vi "Launcher.vi"() -> ()   [LabVIEW 2019, in "Aplicacion.lvclass"]
uses:
  Aplicacion.lvclass
  Pruebas/AjustesPrevios/AjustesPrevios.lvclass
  Equipo/Equipo/Equipo.lvclass
  Equipo/Fabrica de Equipos/Fabrica de Equipos.lvclass
panel:
  in  "Certificado":bool
  in  "Salir":bool
  in  "Ensayos":bool
  in  "Configuraciones":bool
  in  "Usuarios":bool
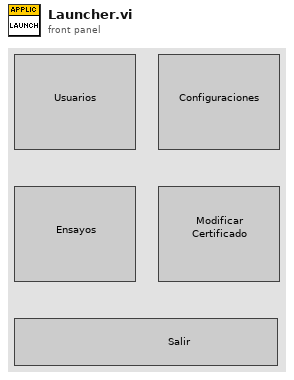
[diagram p1: front panel]
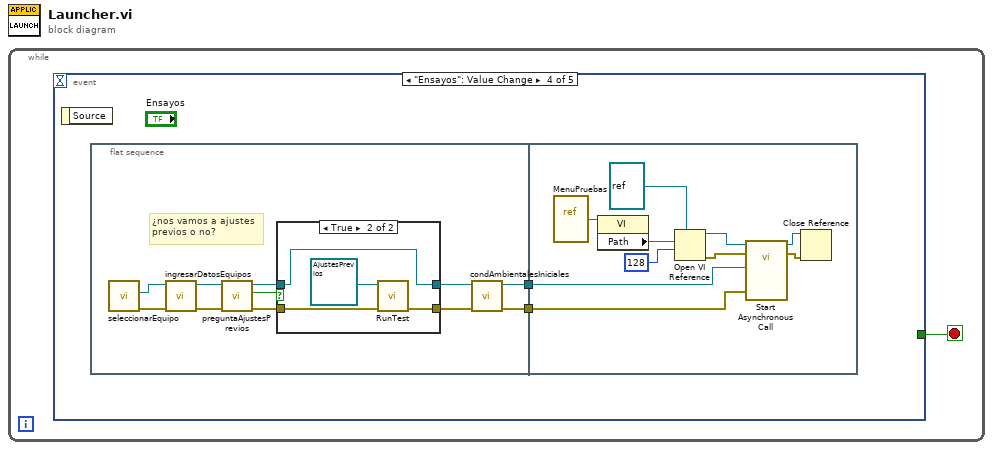
[diagram p0: block diagram]
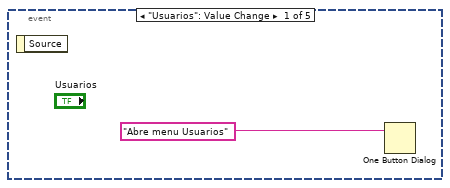
[diagram p2: hidden frame]
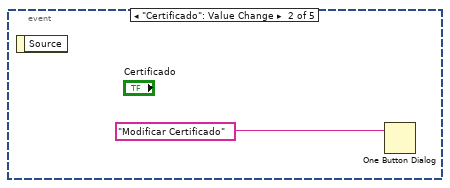
[diagram p3: hidden frame]
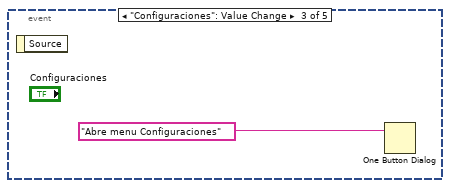
[diagram p4: hidden frame]
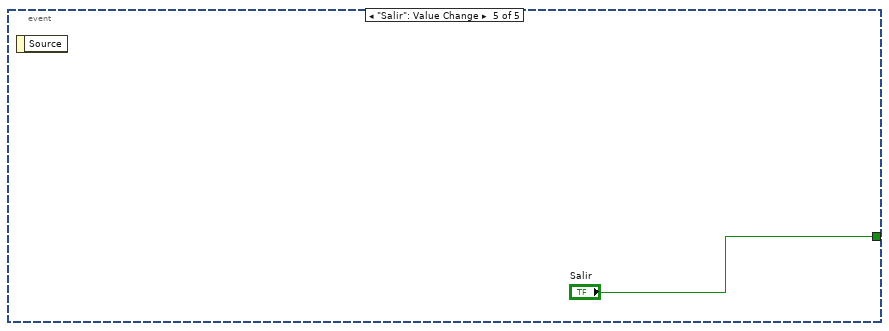
[diagram p6: hidden frame]
diagram:
  n1 = while {
    stop <- w1 stop-if-true
    n2 = event shown="[3] \"Ensayos\": Value Change" {
      selector: _ -> [_ _ _ _ _]
      dyn-events: _ -> [_ _ _ _ _]
      timeout: _ -> [_ _ _ _ _]
      tunnel: [_ _ _ _ "Salir"] -> w1
      event "Usuarios": Value Change {
        n3 = event-data() -> ()  [unwired: 1 in, 1 out]
        n4 = One Button Dialog(message="Abre menu Usuarios") -> ()  [unwired: 1 in, 1 out]
      }
      event "Certificado": Value Change {
        n5 = event-data() -> ()  [unwired: 1 in, 1 out]
        n6 = One Button Dialog(message="Modificar Certificado") -> ()  [unwired: 1 in, 1 out]
      }
      event "Configuraciones": Value Change {
        n7 = event-data() -> ()  [unwired: 1 in, 1 out]
        n8 = One Button Dialog(message="Abre menu Configuraciones") -> ()  [unwired: 1 in, 1 out]
      }
      event "Ensayos": Value Change {
        n9 = event-data() -> ()  [unwired: 1 in, 1 out]
        n10 = flat-sequence {
          tunnel: [w9] -> w6
          tunnel: [w11] -> w5
          tunnel: w6 -> [w25]
          tunnel: w5 -> [w24]
          frame #0 {
            # "¿nos vamos a ajustes\nprevios o no?"
            n11 = call "seleccionarEquipo.vi"() -> ("error out"=w17:errorcluster, "Equipo.lvclass"=w16:refnum<class "Equipo.lvclass">)  [unwired: 9 in, 1 out]
            n12 = call-dynamic "ingresarDatosEquipos.vi"("error in (no error)"=w17, "Equipo in"=w16) -> ("error out"=w7:errorcluster, "Equipo out"=w8:refnum<class "Equipo.lvclass">)  [unwired: 8 in]
            n13 = call "preguntaAjustesPrevios.vi"("error in (no error)"=w7, "Equipo in"=w8) -> ("error out"=w14:errorcluster, "Si"=w12:bool, "Equipo out"=w13:refnum<class "Equipo.lvclass">)  [unwired: 7 in]
            n14 = case shown="True" w12 {
              tunnel: [w19 w23] -> w10
              tunnel: w13 -> [w19 w23]
              tunnel: [w18 w21] -> w15
              tunnel: w14 -> [w18 w22]
              frame False {
              }
              frame True {
                n15 = call-dynamic "RunTest.vi"("error in (no error)"=w22, "AjustesPrevios in"=refnum<class "AjustesPrevios.lvclass"> refnum) -> ("error out"=w21:errorcluster)  [unwired: 7 in, 2 out]
              }
            }
            n16 = call-dynamic "condAmbientalesIniciales.vi"("error in (no error)"=w15, "Equipo in"=w10) -> ("error out"=w11:errorcluster, "Equipo out"=w9:refnum<class "Equipo.lvclass">)  [unwired: 8 in]
          }
          frame #1 {
            n17 = vi-ref "MenuPruebas.vi"() -> (w33:refnum<vi>)
            n18 = property class="VI"(reference=w33) -> ("Path"=w32:path)  [unwired: 1 in, 2 out]
            n19 = Open VI Reference(type specifier VI Refnum (for type only)=refnum<vi> refnum, vi path=w32, options=128) -> (vi reference=w26:refnum<vi>, error out=w30:errorcluster)  [unwired: 3 in]
            n20 = call-by-ref "Start Asynchronous Call"(reference=w26, error in=w30, 8:"error in (no error)"=w24, "Equipo.lvclass"=w25) -> (reference out=w29:refnum<vi>, error out=w28:errorcluster)  [unwired: 9 in, 1 out]
            n21 = Close Reference(reference=w29, error in (no error)=w28) -> ()  [unwired: 1 out]
          }
        }
      }
      event "Salir": Value Change {
        n22 = event-data() -> ()  [unwired: 1 in, 1 out]
      }
    }
  }
